vi "Actor Core.vi"(8 "error in":errorcluster, 11 "CONTADOR_CON_LIMITES in":refnum<class "CONTADOR_CON_LIMITES.lvclass">) -> (0 "error out":errorcluster, 3 "Actor out":refnum<class "Actor.lvclass">)   [LabVIEW 2019, in "CONTADOR_CON_LIMITES.lvlib" / "CONTADOR_CON_LIMITES.lvclass"]
doc: "(<B>Filename</B>: Actor Framework.lvlib:Actor.lvclass:Actor Core.vi)\n\nReceives messages to the actor, reacts to them, and initiates any error handling that may shut the actor down.\n\nDescendant classes may override this VI to append parallel tasks for the actor to complete while it handles messages. Overrides use the Call Parent Method node."
uses:
  CONTADOR_CON_LIMITES.lvclass
  C:/Program Files (x86)/National Instruments/LabVIEW 2019/vi.lib/ActorFramework/Actor/Actor.lvclass
  <vilib>/ActorFramework/Actor/Actor.lvclass
  <vilib>/ActorFramework/Actor/Actor.lvclass/Actor.ctl
  CONTADOR_CON_LIMITES.lvclass/CONTADOR_CON_LIMITES.ctl
panel:
  out "LÍMITE INFERIOR 2":dbl
  out "LÍMITE SUPERIOR 2":dbl
  out "LÍMITE INFERIOR":dbl
  out "NUMERO ACTUAL":dbl
  out "START/STOP HL":bool
  out "LÍMITE SUPERIOR":dbl
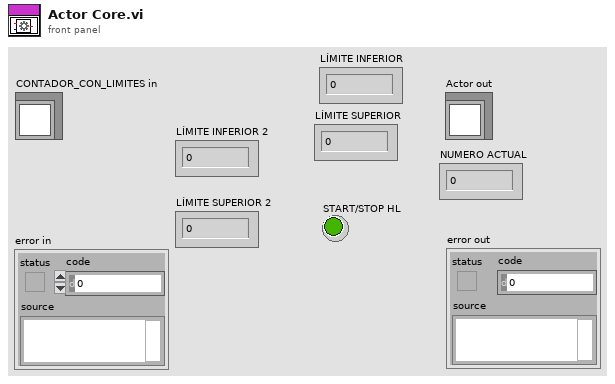
[diagram p1: front panel]
types:
  T1 = cluster{"LÍMITE SUPERIOR":dbl, "LÍMITE INFERIOR":dbl, "NUMERO ACTUAL":dbl}
  T2 = cluster{"START/STOP EVENT":refnum<user-event>, "LIMITES EVENT":refnum<user-event>, "EXIT EVENT":refnum<user-event>}
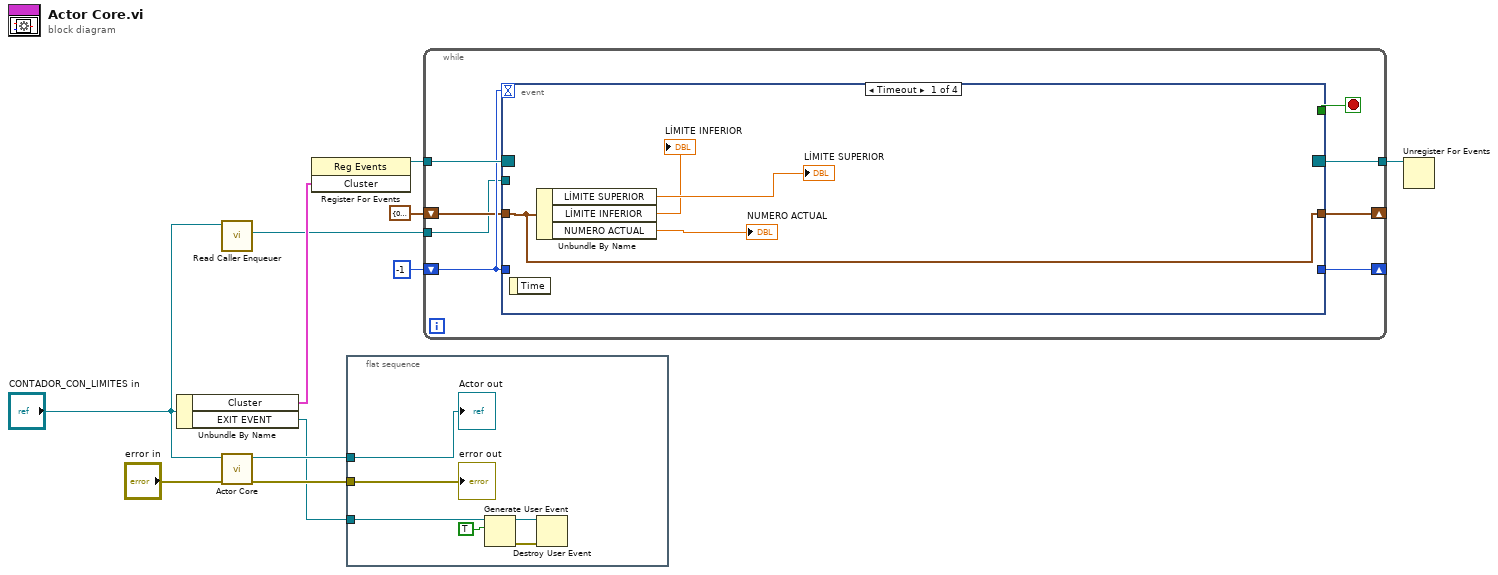
[diagram p0: block diagram]
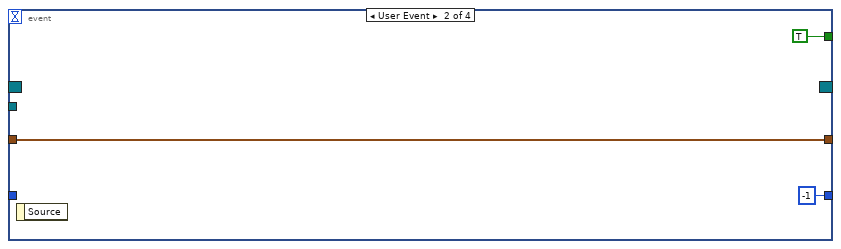
[diagram p2: hidden frame]
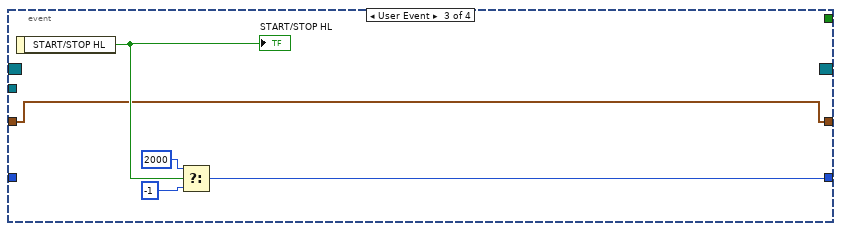
[diagram p3: hidden frame]
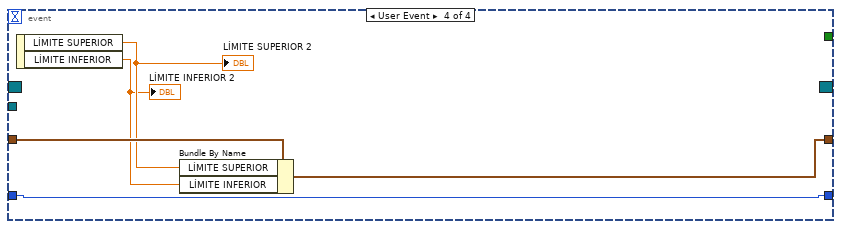
[diagram p4: hidden frame]
diagram:
  n1 = Unbundle By Name("CONTADOR_CON_LIMITES in") -> ("Cluster"=w8:T2, "EXIT EVENT"=w5:refnum<user-event>)
  n2 = call <vilib>:"Read Caller Enqueuer.vi"("Actor"="CONTADOR_CON_LIMITES in") -> ("Caller Enqueuer"=w2:refnum<class "Message Enqueuer.lvclass">)  [unwired: 10 in]
  n3 = call-parent "Actor Core.vi"("error in"="error in", "Actor in"="CONTADOR_CON_LIMITES in") -> ("error out"=w11:errorcluster, "Actor out"=w10:refnum<class "Actor.lvclass">)  [unwired: 8 in]
  n4 = register-events(w8) -> (reference out=w7:refnum<event-registration>)  [unwired: 2 in, 1 out]
  n5 = flat-sequence {
    tunnel: w11 -> [w17]
    tunnel: w10 -> [w16]
    tunnel: w5 -> [w15]
    frame #0 {
      n6 = Generate User Event(user event=w15, event data cluster=TRUE ("event data")) -> (user event out=w12:refnum<user-event>, error out=w13:errorcluster)  [unwired: 2 in]
      n7 = Destroy User Event(user event=w12, error in=w13) -> ()  [unwired: 1 out]
      "error out" <- w17
      "Actor out" <- w16
    }
  }
  n8 = while {
    tunnel: w7 -> [w25]
    tunnel: [w24] -> w6
    shift-right: [w22] -> _
    shift-left: -1 ("f") -> [w21]
    shift-right: [w19] -> _
    shift-left: T1 {"LÍMITE SUPERIOR"=0.0, "LÍMITE INFERIOR"=0.0, "NUMERO ACTUAL"=0.0} -> [w20]
    tunnel: w2 -> [w18]
    stop <- w23 stop-if-true
    n9 = event shown="[0] Timeout" {
      selector: w25 -> [_ _ _ _]
      dyn-events: [_ _ _ _] -> w24
      timeout: w21 -> [_ _ _ _]
      tunnel: [_ TRUE _ _] -> w23
      tunnel: [_ -1 ("f") w34 w38] -> w22
      tunnel: w21 -> [_ _ _ w38]
      tunnel: w20 -> [w26 w31 w33 w42]
      tunnel: [w26 w31 w33 w39] -> w19
      tunnel: w18 -> [_ _ _ _]
      event Timeout {
        n10 = event-data() -> ()  [unwired: 1 in, 1 out]
        n11 = Unbundle By Name(w26) -> ("LÍMITE SUPERIOR"=→"LÍMITE SUPERIOR":dbl, "LÍMITE INFERIOR"=→"LÍMITE INFERIOR":dbl, "NUMERO ACTUAL"=→"NUMERO ACTUAL":dbl)
      }
      event User Event {
        n12 = event-data() -> ()  [unwired: 1 in, 1 out]
      }
      event User Event {
        n13 = event-data() -> ("START/STOP HL"=w37:bool)  [unwired: 1 in]
        "START/STOP HL" <- w37
        n14 = Select(t=2000, s=w37, f=-1) -> (s? t:f=w34:i32)
      }
      event User Event {
        n15 = event-data() -> ("LÍMITE SUPERIOR"=w41:dbl, "LÍMITE INFERIOR"=w40:dbl)  [unwired: 1 in]
        "LÍMITE SUPERIOR 2" <- w41
        "LÍMITE INFERIOR 2" <- w40
        n16 = Bundle By Name(cluster=w42, "LÍMITE SUPERIOR"=w41, "LÍMITE INFERIOR"=w40) -> (w39:T1)
      }
    }
  }
  n17 = Unregister For Events(event registration refnum=w6) -> ()  [unwired: 1 in, 1 out]
